vi "SPC_set_page.vi"(8 "Error In":errorcluster, 9 "Page":i32 min=0 max=65535 step=1, 10 "Module No":i16=-1 min=-1 max=7 step=1, 11 "DLL Path":path) -> (0 "Error Out":errorcluster, 1 "Page":i32, 2 "Module No":i16, 3 "DLL Path":path)   [LabVIEW 2017]
doc: "The procedure defines the page of memory (on SPC module ‘mod_no’) in which the data of a subsequent measurement will be recorded. SPC_set_page must be called before a measurement is started.\nIf ‘mod_no’ = -1, page will be changed for all SPC modules which are actually in use. Be sure that in such case all modules are configured in the same way (the best is to use SPC_configure_memory with ‘mod_no’ = -1).\nThe range of the parameters ‘block’ and ‘page’ depends on the actual configuration of the SPC memory (see SPC_configure_memory). To provide correct access to the SPC memory it is required that the function SPC_configure_memory be used before the first call of SPC_set_page ( in normal modes). This function also delivers the required information about the block/page structure of the SPC memory:\nlong max_block_no total number of blocks (=curves) in the memory ( memory bank for the SPC-6x0/13x/15x/160)\nlong blocks_per_frame Number of blocks (=curves) per frame\nlong frames_per_page Number of frames per page\nlong maxpage max number of pages to use in a measurement\nlong block_length Number of 16-bits words per one block (curve)\n\ninfo@becker-hickl.com"
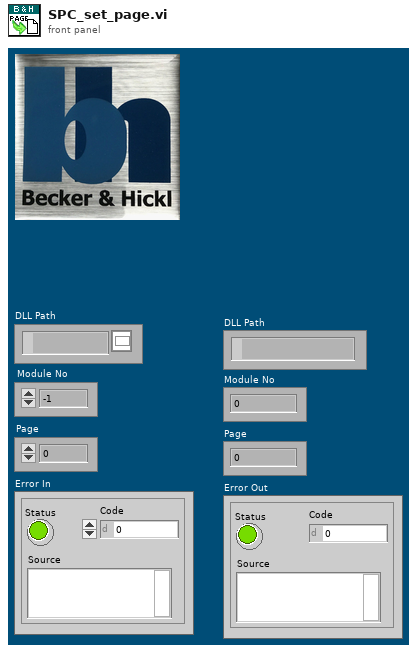
[diagram p1: front panel]
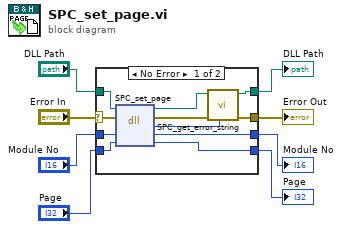
[diagram p0: block diagram]
diagram:
  n1 = case shown="No Error" "Error In" {
    selector: "Error In" -> [w18 w22]
    tunnel: "DLL Path" -> [w19 w23]
    tunnel: [w12 w23] -> w7
    tunnel: [w11 w22] -> w6
    tunnel: "Module No" -> [w17 w21]
    tunnel: [w16 w21] -> w3
    tunnel: [w15 w20] -> w2
    tunnel: "Page" -> [w14 w20]
    frame No Error {
      n2 = dll-call lib="D:/spcm/lib/lab_view/lv10.0/spcm32.dll" fn="SPC_set_page"(path in=w19, error in=w18, "mod_no"=w17, "page"=w14) -> (path out=w13:path, error out=w10:errorcluster, "return type"=w9:i16, "mod_no"=w16:i16, "page"=w15:i32)  [unwired: 1 in]
      n3 = call "SPC_get_error_string.vi"("ErrorID"=w9, "Error In"=w10, "DLL Path"=w13) -> ("Error Out"=w11:errorcluster, "DLL Path"=w12:path)  [unwired: 6 in, 1 out]
    }
    frame Error {
    }
  }
  "DLL Path" <- w7
  "Error Out" <- w6
  "Module No" <- w3
  "Page" <- w2
